vi "Get DB Data.vi"(8 "error in (no error)":errorcluster caption="에러 입력(에러 없음)", 10 "SQL query":string, 11 "connection reference":T1) -> (0 "error out":errorcluster caption="에러 출력", 1 "No":i32[](array[numeric]), 2 "Data":string[][](array[string]), 3 "connection reference":T1, 4 "None?":bool)   [LabVIEW 2020]
uses:
  <vilib>/addons/database/Connection.llb/Conn ObjectReference.ctl
  <vilib>/addons/database/Connection.llb/Conn Execute.vi
  <vilib>/addons/database/Recordset.llb/Rec Get Recordset Properties (R).vi
  <vilib>/addons/database/Recordset.llb/Rec Fetch Recordset Data (R).vi
  <vilib>/addons/database/Recordset.llb/Rec Destroy - Connection.vi
  <vilib>/addons/database/_DB Variant To Data/Database Variant To Data.xnode
  <vilib>/addons/database/NI_Database_API.lvlib
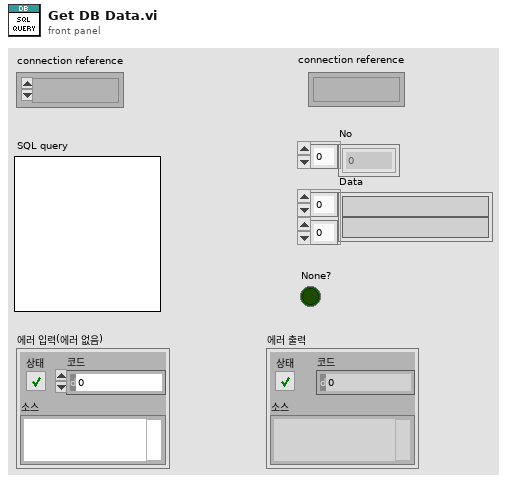
[diagram p1: front panel]
types:
  T1 = typedef "NI_Database_API.lvlib/Conn ObjectReference.ctl" = refnum<k1>
  T2 = typedef "NI_Database_API.lvlib/Rec ObjectReference.ctl" = refnum<k1>
  T3 = typedef "NI_Database_API.lvlib/Rec Properties.ctl" = cluster{"column count":i32, "record index":i32, "record count":i32, "bof?":bool, "eof?":bool, "cursor type":T4, "cache size":i32, "state":enum16{"closed", "open"}}
  T4 = typedef "NI_Database_API.lvlib/DB Tools Cursor Type.ctl" = enum16{"forward-only", "keyset", "dynamic", "static"}
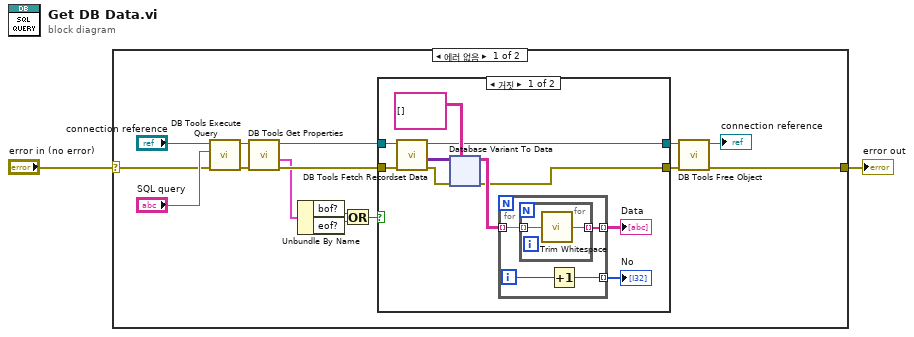
[diagram p0: block diagram]
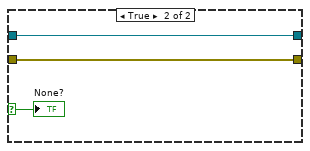
[diagram p2: hidden frame]
diagram:
  n1 = case shown="에러 없음" "error in (no error)" {
    selector: "error in (no error)" -> [w15 w81]
    tunnel: [w4 w81] -> w2
    frame No Error {
      n2 = call-poly <vilib>:"DB Tools Execute Query.vi"("error in (no error)"=w15, "SQL query"="SQL query", "connection reference"="connection reference") -> ("error out"=w14:errorcluster, "recordset reference"=w12:T2)  [unwired: 5 in]
      n3 = call-poly <vilib>:"DB Tools Get Properties.vi"("error in (no error)"=w14, "recordset reference"=w12) -> ("error out"=w13:errorcluster, "recordset properties"=w10:T3, "recordset reference out"=w11:T2)  [unwired: 3 in]
      n4 = Unbundle By Name(w10) -> ("bof?"=w9:bool, "eof?"=w8:bool)
      n5 = Or(x=w9, y=w8) -> (x .or. y?=w7:bool)
      n6 = case shown="거짓" w7 {
        selector: w7 -> [_ w78]
        tunnel: w13 -> [w21 w79]
        tunnel: w11 -> [w20 w80]
        tunnel: [w19 w80] -> w6
        tunnel: [w18 w79] -> w3
        frame False {
          n7 = call-poly <vilib>:"DB Tools Fetch Recordset Data.vi"("error in (no error)"=w21, "recordset reference"=w20) -> ("error out"=w25:errorcluster, "recordset data"=w27:variant[][], "recordset reference out"=w19:T2)  [unwired: 3 in]
          n8 = xnode "Database Variant To Data"("database variant"=w27, "error in (no error)"=w25, "type"=string[][] []) -> ("data"=w24:string[][], "error out"=w18:errorcluster)
          n9 = for {
            tunnel: w24 -> [w31] mode=indexing
            tunnel: [w30] -> w23 mode=indexing
            tunnel: [w28] -> w22 mode=indexing
            i -> [w29]
            n10 = for {
              tunnel: w31 -> [w33] mode=indexing
              tunnel: [w32] -> w30 mode=indexing
              n11 = call <vilib>:"Trim Whitespace.vi"("string"=w33) -> ("trimmed string"=w32:string)  [unwired: 1 in]
            }
            n12 = Increment(x=w29) -> (x+1=w28:i32)
          }
          "Data" <- w23
          "No" <- w22
        }
        frame True {
          "None?" <- w78
        }
      }
      n13 = call-poly <vilib>:"DB Tools Free Object.vi"("error in (no error)"=w3, "recordset reference"=w6) -> ("error out"=w4:errorcluster, "connection reference"=→"connection reference":T1)  [unwired: 8 in]
    }
    frame Error {
    }
  }
  "error out" <- w2
